vi "Set Gate.vi"(8 "error in (no error)":errorcluster, 9 "stepRenamed":sgl, 10 "width":sgl, 11 "delay":sgl) -> (0 "error out":errorcluster, 3 "function return":u32)   [LabVIEW 2014, in "atmcd32d.lvlib"]
doc: "unsigned int WINAPI SetGate(float delay, float width, float stepRenamed);"
uses:
  atmcd32d.lvlib
  atmcd32d.dll
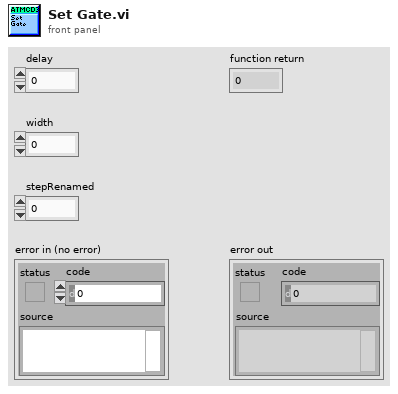
[diagram p1: front panel]
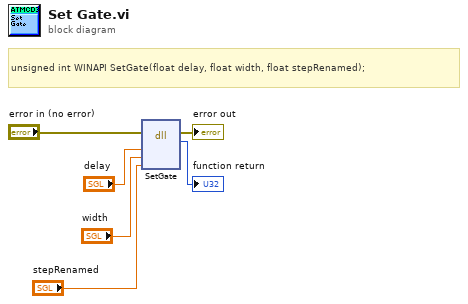
[diagram p0: block diagram]
diagram:
  # "unsigned int WINAPI SetGate(float delay, float width, float stepRenamed);"
  n1 = dll-call lib="C:/Users/Bakir/Documents/Lambda2-Testing/lib/Andorlib/atmcd32d.*" fn="SetGate"(error in="error in (no error)", "delay"="delay", "width"="width", "stepRenamed"="stepRenamed") -> (error out=→"error out":errorcluster, →"function return":u32)  [unwired: 5 in, 1 out]
